vi "10.4 Create Files and Folders.vi"() -> ()   [LabVIEW 2019]
uses:
  <vilib>/Utility/sysdir.llb/System Directory Type.ctl
panel:
  in  "Selector":T1(ring)
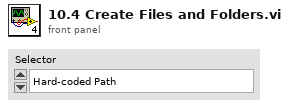
[diagram p1: front panel]
types:
  T1 = enum16{"Hard-coded Path", "File Dialog", "Current VI Folder Path", "System Folder Path"}
  T2 = enum16{"open", "replace", "create", "open or create", "replace or create", "replace or create with confirmation"}
  T3 = typedef "System Directory Type.ctl" = i32
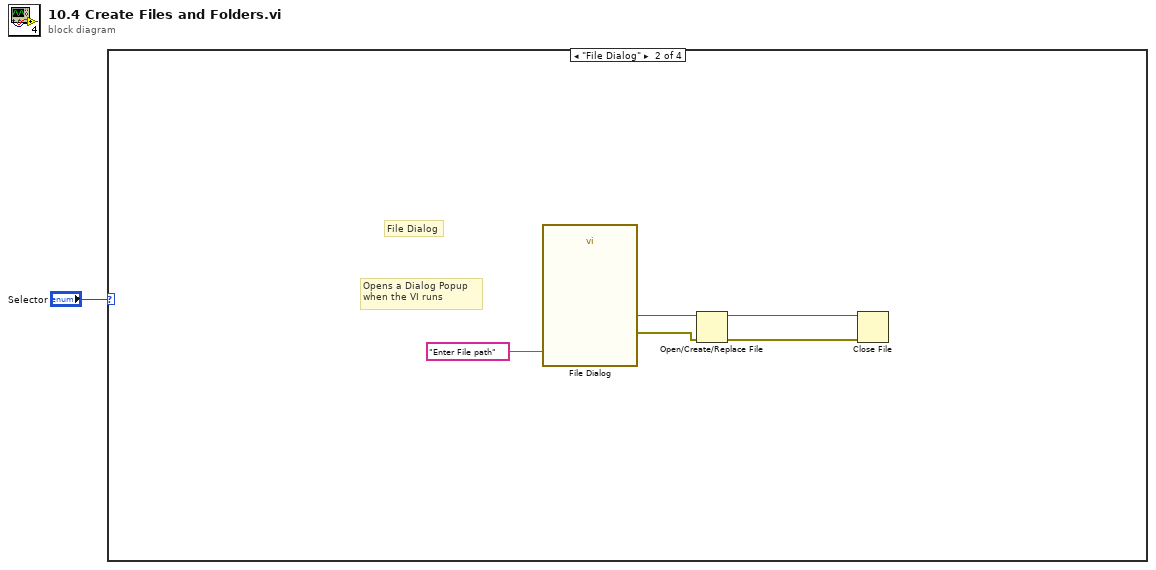
[diagram p0: block diagram]
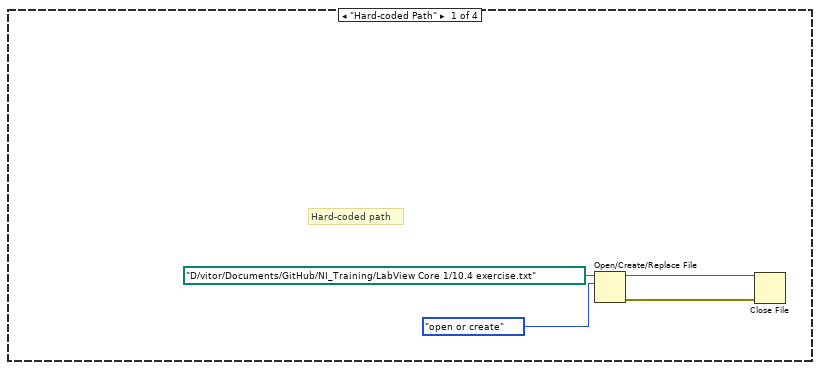
[diagram p2: hidden frame]
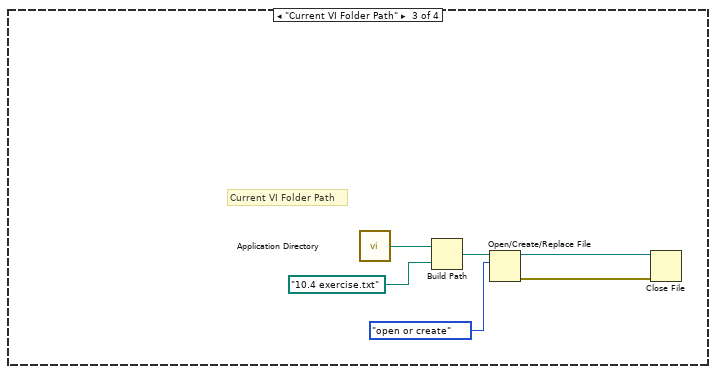
[diagram p3: hidden frame]
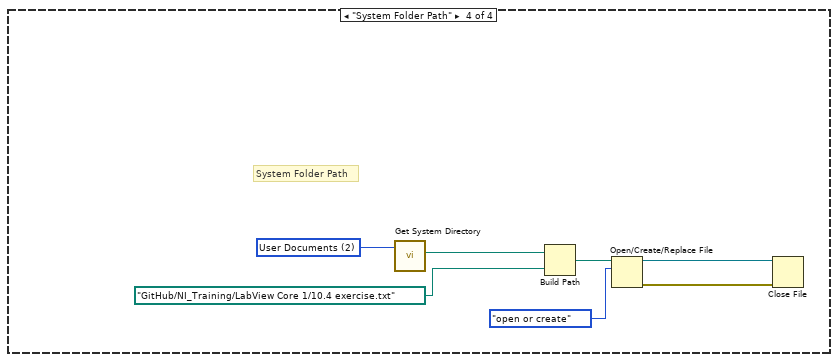
[diagram p4: hidden frame]
diagram:
  n1 = case shown="\"File Dialog\"" "Selector" {
    frame "Hard-coded Path" {
      # "Hard-coded path"
      n2 = Open/Create/Replace File(file path (use dialog)=path "D:/vitor/Documents/GitHub/NI_Training/LabView Core 1/10.4 exercise.txt", operation (0:open)=T2."open or create") -> (refnum out=w4:refnum<file>, error out=w5:errorcluster)  [unwired: 4 in, 1 out]
      n3 = Close File(refnum=w4, error in=w5) -> ()  [unwired: 2 out]
    }
    frame "File Dialog" {
      # "Opens a Dialog Popup\nwhen the VI runs"
      # "File Dialog"
      n4 = call "File Dialog"("prompt"="Enter File path") -> ("selected path"=w7:path, "error out"=w8:errorcluster)  [unwired: 11 in, 2 out]
      n5 = Open/Create/Replace File(file path (use dialog)=w7, error in=w8) -> (refnum out=w9:refnum<file>, error out=w10:errorcluster)  [unwired: 4 in, 1 out]
      n6 = Close File(refnum=w9, error in=w10) -> ()  [unwired: 2 out]
    }
    frame "Current VI Folder Path" {
      # "Current VI Folder Path"
      n7 = call <vilib>:"Application Directory.vi"() -> ("Application Directory"=w13:path)
      n8 = Build Path(base path=w13, name or relative path=path "10.4 exercise.txt") -> (appended path=w16:path)
      n9 = Open/Create/Replace File(file path (use dialog)=w16, operation (0:open)=T2."open or create") -> (refnum out=w15:refnum<file>, error out=w14:errorcluster)  [unwired: 4 in, 1 out]
      n10 = Close File(refnum=w15, error in=w14) -> ()  [unwired: 2 out]
    }
    frame "System Folder Path" {
      w18 = T3 2 items=["User Home"=0, "User Desktop"=1, "User Documents"=2, "User Application Data"=3, "User Preferences"=4, "User Temporary"=5, "Public Documents"=6, "Public Application Data"=7, "Public Preferences"=8, "Public Cache"=13, "System Core Libraries"=9, "System Installed Libraries"=10, "Application Files"=11, "Boot Volume Root"=12] ("system directory type")
      # "System Folder Path"
      n11 = call <vilib>:"Get System Directory.vi"("system directory type"=w18) -> ("system directory"=w23:path)  [unwired: 10 in]
      n12 = Build Path(base path=w23, name or relative path=path "GitHub/NI_Training/LabView Core 1/10.4 exercise.txt") -> (appended path=w20:path)
      n13 = Open/Create/Replace File(file path (use dialog)=w20, operation (0:open)=T2."open or create") -> (refnum out=w21:refnum<file>, error out=w22:errorcluster)  [unwired: 4 in, 1 out]
      n14 = Close File(refnum=w21, error in=w22) -> ()  [unwired: 2 out]
    }
  }
